vi "Template - Function Generator Software Triggered Frequency Sweep.vi"() -> ()   [LabVIEW 2020]
doc: "This example shows how to configure and enable a triggered frequency sweep."
uses:
  <instrlib>/_Template - Function Generator/Template - Function Generator.lvlib
panel:
  in  "Waveform Function (0: Sine)":u16(ring) items=["Sine", "Square", "Triangle"]
  in  "Serial Configuration":T1={"Baud Rate"=9600, "Parity"=0, "Data Bits"=7, "Stop Bits"=10, "Flow Control"=0} {"Flow Control" items=["None", "XON/XOFF", "RTS/CTS", "XON/XOFF & RTS/CTS", "DTR/DSR", "XON/XOFF & DTR/DSR"]; "Stop Bits" items=["1.0"=10, "1.5"=15, "2.0"=20]; "Data Bits" items=["7"=7, "8"=8]; "Parity" items=["None", "Odd", "Even", "Mark", "Space"]; "Baud Rate" items=["300"=300, "600"=600, "1200"=1200, "2400"=2400, "4800"=4800, "9600"=9600, "19200"=19200]}
  in  "Stop  Frequency  (1000.0 Hz)":dbl=1000.0 format="%#.6g"
  in  "Start Frequency (100.0 Hz)":dbl=100.0 format="%#.6g"
  in  "Sweep Time (1.00 s)":dbl=1.0 format="%#.6g"
  in  "Amplitude (0.1 Vpp)":dbl=0.1
  in  "VISA resource name":refnum<visa-resource-name>
  # "(c) 2014 <Enter Company Name Here>.  ALL RIGHTS RESERVED."
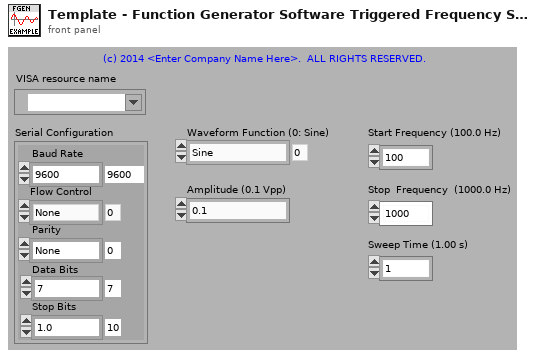
[diagram p1: front panel]
types:
  T1 = cluster{"Baud Rate":u32, "Parity":u16, "Data Bits":u16, "Stop Bits":u16, "Flow Control":u16}
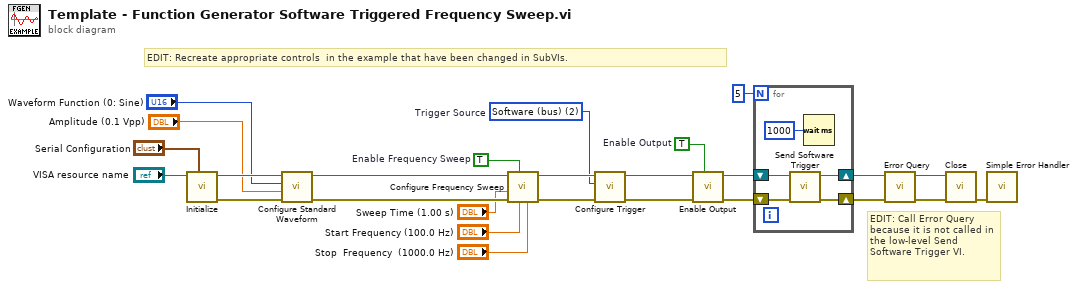
[diagram p0: block diagram]
diagram:
  w2 = TRUE  # Enable Output
  w13 = u16 2 items=["Internal", "External", "Software (bus)"]  # Trigger Source
  w20 = TRUE  # Enable Frequency Sweep
  # "EDIT: Call Error Query because it is not called in the low-level Send Software Trigger VI."
  # "EDIT: Recreate appropriate controls  in the example that have been changed in SubVIs."
  n1 = call <instrlib>:"Initialize.vi"("Serial Configuration"="Serial Configuration", "VISA resource name"="VISA resource name") -> ("error out"=w21:errorcluster, "VISA resource name out"=w26:refnum<visa-resource-name>)  [unwired: 8 in]
  n2 = call <instrlib>:"Configure Standard Waveform.vi"("error in (no error)"=w21, "Amplitude (1.0 Vpp)"="Amplitude (0.1 Vpp)", "Waveform Function (0: Sine)"="Waveform Function (0: Sine)", "VISA resource name"=w26) -> ("error out"=w24:errorcluster, "VISA resource name out"=w23:refnum<visa-resource-name>)  [unwired: 6 in]
  n3 = call <instrlib>:"Configure Frequency Sweep.vi"("Stop  Frequency  (1000.0 Hz)"="Stop  Frequency  (1000.0 Hz)", "Start Frequency (100.0 Hz)"="Start Frequency (100.0 Hz)", "Enable Frequency Sweep (T:Enable)"=w20, "error in (no error)"=w24, "Sweep Time (1.00 s)"="Sweep Time (1.00 s)", "VISA resource name"=w23) -> ("error out"=w18:errorcluster, "VISA resource name out"=w19:refnum<visa-resource-name>)  [unwired: 4 in]
  n4 = call <instrlib>:"Configure Trigger.vi"("error in (no error)"=w18, "Trigger Source (0: Internal)"=w13, "VISA resource name"=w19) -> ("error out"=w17:errorcluster, "VISA resource name out"=w16:refnum<visa-resource-name>)  [unwired: 7 in]
  n5 = call <instrlib>:"Enable Output.vi"("Enable Output (T: Enable)"=w2, "error in (no error)"=w17, "VISA resource name"=w16) -> ("error out"=w8:errorcluster, "VISA resource name out"=w15:refnum<visa-resource-name>)  [unwired: 7 in]
  n6 = for {
    N: 5 -> [_]
    shift-right: [w29] -> w4
    shift-left: w8 -> [w27]
    shift-right: [w30] -> w6
    shift-left: w15 -> [w31]
    n7 = call <instrlib>:"Send Software Trigger.vi"("error in (no error)"=w27, "VISA resource name"=w31) -> ("error out"=w29:errorcluster, "VISA resource name out"=w30:refnum<visa-resource-name>)  [unwired: 8 in]
    n8 = Wait (ms)(milliseconds to wait=u32 1000 ("millisecond multiple")) -> ()  [unwired: 1 out]
  }
  n9 = call <instrlib>:"Error Query.vi"("error in (no error)"=w4, "VISA resource name"=w6) -> ("error out"=w3:errorcluster, "VISA resource name out"=w5:refnum<visa-resource-name>)  [unwired: 6 in, 2 out]
  n10 = call <instrlib>:"Close.vi"("error in (no error)"=w3, "VISA resource name"=w5) -> ("error out"=w25:errorcluster)  [unwired: 9 in]
  n11 = call <vilib>:"Simple Error Handler.vi"("error in (no error)"=w25) -> ()  [unwired: 4 in, 5 out]
